vi "Target Dataset.vi"(8 "error in (no error)":errorcluster, 10 "Current Target In":T1[](array[typedef]), 11 "Mixed Mode Commands\n Datastore Actions":T2) -> (0 "error out":errorcluster, 3 "Current Target Out":T1[](array[typedef]))   [LabVIEW 2009]
uses:
  Data Access Objects/Metadata/DAO Actions.ctl
  MixedMode/Target Data.ctl
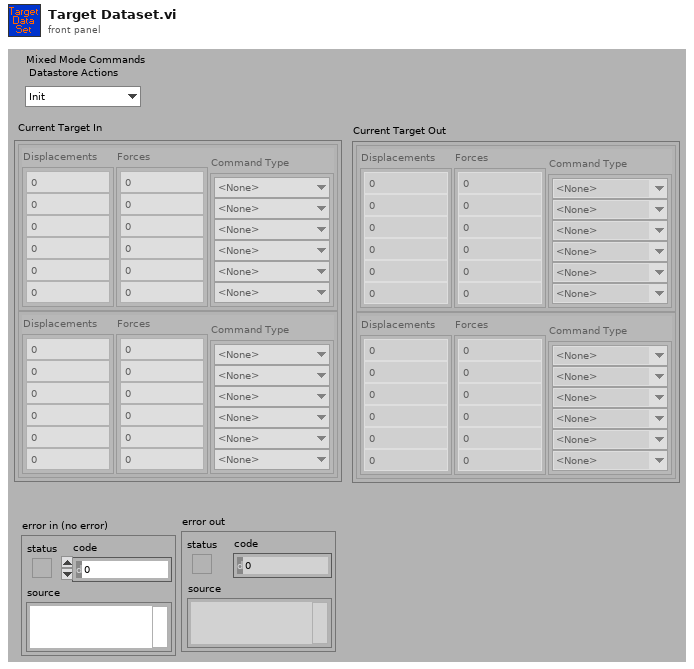
[diagram p1: front panel]
types:
  T1 = typedef "Target Data.ctl" = cluster{"Displacements":dbl[], "Command Type":enum16{"<None>", "Displacement", "Force"}[], "Forces":dbl[]}
  T2 = typedef "DAO Actions.ctl" = enum16{"Init", "Get", "Set"}
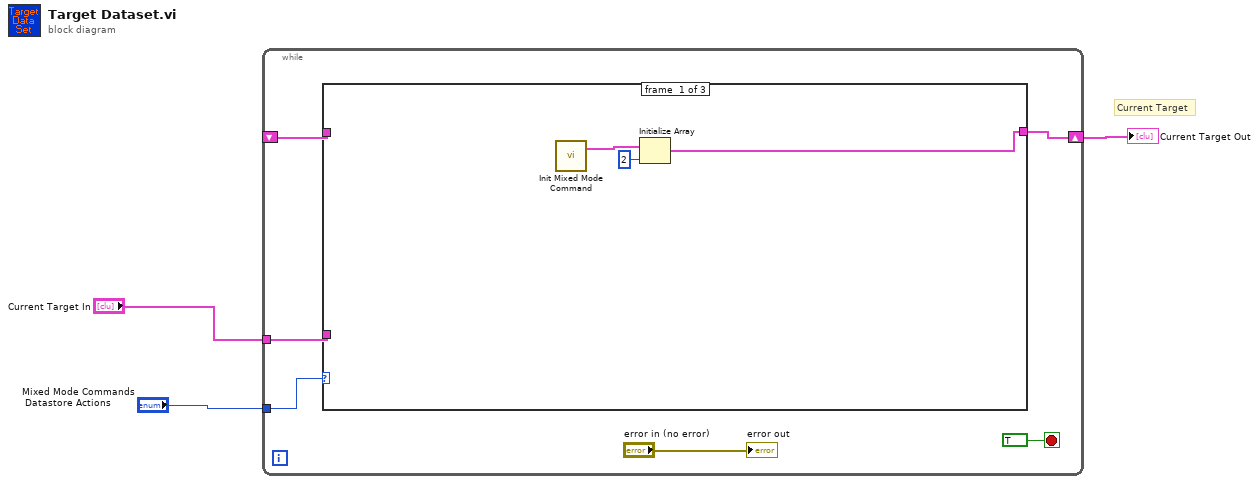
[diagram p0: block diagram]
diagram:
  # "Current Target"
  n1 = while {
    tunnel: "Mixed Mode Commands\n Datastore Actions" -> [w9]
    shift-right: [w7] -> w1
    shift-left: _ -> [w6]
    tunnel: "Current Target In" -> [w5]
    stop <- TRUE stop-if-true
    n2 = case shown="\"Set\"" w9 {
      tunnel: [w11 w13 w14] -> w7
      tunnel: w6 -> [_ _ w14]
      tunnel: w5 -> [_ w13 _]
      frame #0 {
        n3 = call "Init Mixed Mode Command.vi"() -> ("Command Data"=w12:T1)  [unwired: 1 in, 2 out]
        n4 = Initialize Array(w12, 2 ("dimension size")) -> (w11:T1[])
      }
      frame #1 {
      }
      frame #2 {
      }
    }
    "error out" <- "error in (no error)"
  }
  "Current Target Out" <- w1
